vi "subvi_Calculate_RPM.vi"(8 "에러 입력":errorcluster caption="에러 입력(에러 없음)", 9 "data":waveform(dbl)[](array[waveform]), 11 "Tach CH":i32) -> (0 "에러 출력":errorcluster, 3 "RPM":dbl)   [LabVIEW 2016]
uses:
  <vilib>/measure/mascope.llb/Pulse Measurements 1 chan.vi
  <vilib>/measure/NI_MAPro.lvlib
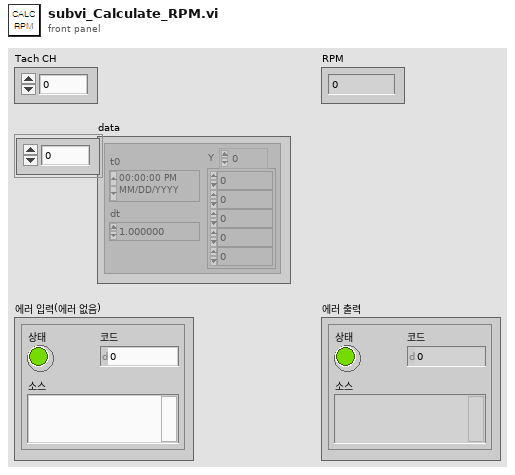
[diagram p1: front panel]
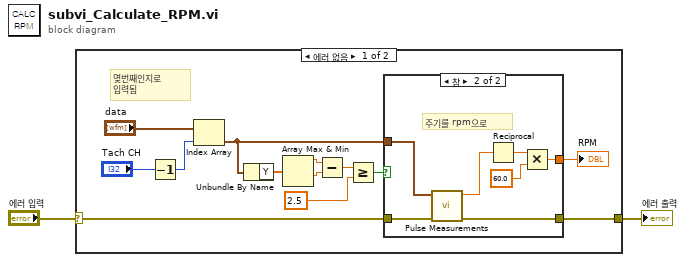
[diagram p0: block diagram]
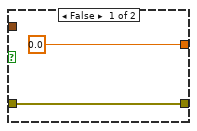
[diagram p2: hidden frame]
diagram:
  n1 = case shown="에러 없음" "에러 입력" {
    selector: "에러 입력" -> [w13 w25]
    tunnel: [w12 w25] -> w1
    frame No Error {
      # "몆번째인지로 \n입력됨"
      n2 = Decrement(x="Tach CH") -> (x-1=w10:i32)
      n3 = Index Array(array="data", index=w10) -> (element=w9:waveform(dbl))
      n4 = Unbundle By Name(w9) -> ("Y"=w8:dbl[])
      n5 = Array Max & Min(array=w8) -> (max value=w7:dbl, min value=w6:dbl)  [unwired: 2 out]
      n6 = Subtract(x=w7, y=w6) -> (x-y=w5:dbl)
      n7 = Greater Or Equal?(x=w5, y=2.5) -> (x >= y?=w3:bool)
      n8 = case shown="참" w3 {
        tunnel: [0.0 w24] -> w14
        tunnel: w9 -> [_ w23]
        tunnel: w13 -> [w17 w22]
        tunnel: [w17 w21] -> w12
        frame False {
        }
        frame True {
          # "주기를 rpm으로"
          n9 = call-poly <vilib>:"Pulse Measurements.vi"("error in (no error)"=w22, "signal in"=w23) -> ("error out"=w21:errorcluster, "period"=w18:dbl)  [unwired: 5 in, 3 out]
          n10 = Reciprocal(x=w18) -> (1/x=w19:dbl)
          n11 = Multiply(x=w19, y=60.0) -> (x*y=w24:dbl)
        }
      }
      "RPM" <- w14
    }
    frame Error {
    }
  }
  "에러 출력" <- w1
